vi "Simulation Interface.vi"(8 "error in (no error)":errorcluster) -> (0 "error out":errorcluster)   [LabVIEW 2017]
doc: "The simulated modules used to validate the Elevator Controller logic and algorithms."
uses:
  View Model/Controls/Interface.ctl
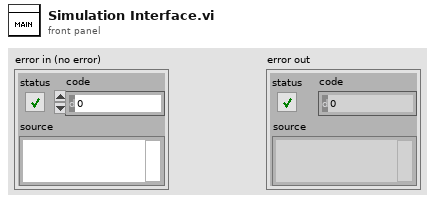
[diagram p1: front panel]
types:
  T1 = typedef "View Model.ctl" = cluster{"Shared Model":T2, "Error Model":T3, "Config Model":T4, "Control Model":T5}
  T2 = typedef "Shared Model.ctl" = cluster{"Stop":refnum<user-event>, "Stop DVR":refnum<data-value>}
  T3 = typedef "Error Model.ctl" = cluster{"Error":refnum<user-event>}
  T4 = typedef "Config Model.ctl" = cluster{"Data DVR":refnum<data-value>, "Config CMD":refnum<user-event>}
  T5 = typedef "Control Model.ctl" = cluster{"Location Change":refnum<user-event>, "Direction Change":refnum<user-event>, "Door Posit Change":refnum<user-event>, "Emergency Change":refnum<user-event>, "Status Change":refnum<user-event>, "Command":refnum<user-event>, "Overhaed DVR":refnum<data-value>}
  T6 = typedef "Interface.ctl" = enum16{"Simulated", "Physical"}
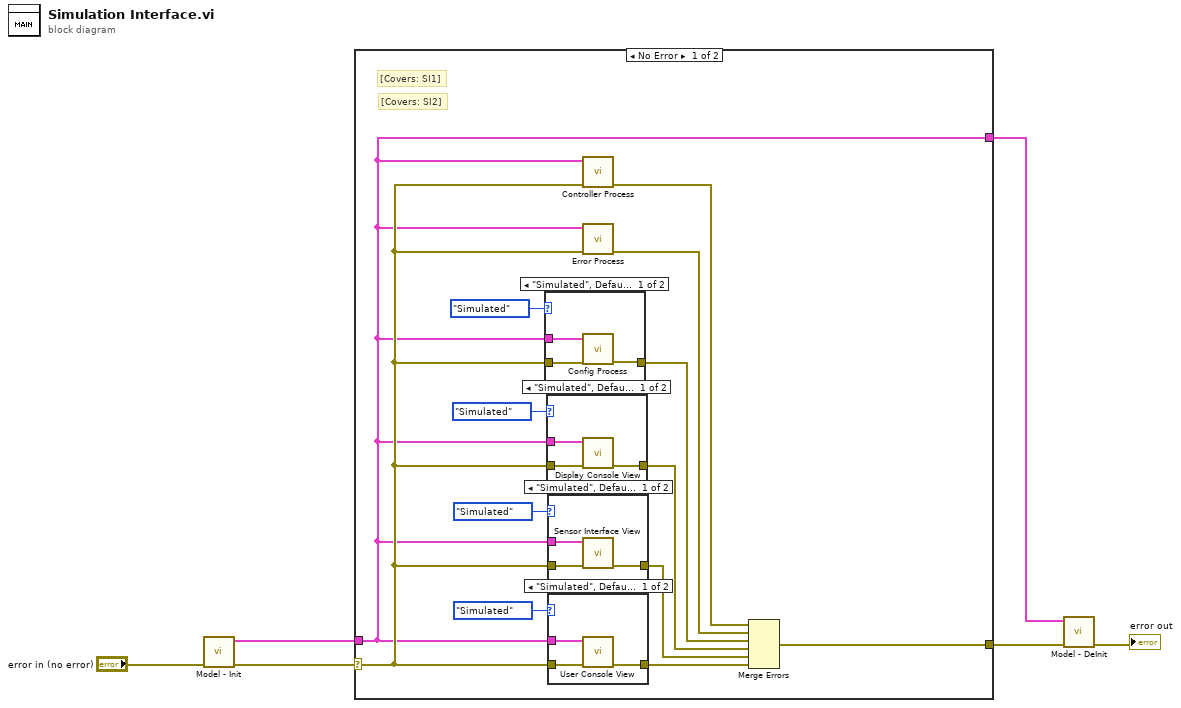
[diagram p0: block diagram]
diagram:
  n1 = call "Model - Init.vi"("error in (no error)"="error in (no error)") -> ("error out"=w4:errorcluster, "View Model"=w5:T1)  [unwired: 9 in]
  n2 = case shown="No Error" w4 {
    selector: w4 -> [w15 w37]
    tunnel: w5 -> [w7 w36]
    tunnel: [w8 w37] -> w3
    tunnel: [w7 w36] -> w1
    frame No Error {
      # "[Covers: SI2]"
      # "[Covers: SI1]"
      n3 = case shown="\"Simulated\", Default" Interface."Simulated" ("Interface") {
        tunnel: w7 -> [w21 _]
        tunnel: w15 -> [w22 w23]
        tunnel: [w20 w23] -> w11
        frame "Simulated", Default {
          n4 = call "Config Process.vi"("error in (no error)"=w22, "View Model"=w21) -> ("error out"=w20:errorcluster)  [unwired: 9 in]
        }
        frame "Physical" {
        }
      }
      n5 = case shown="\"Simulated\", Default" Interface."Simulated" ("Interface") {
        tunnel: w7 -> [w24 _]
        tunnel: w15 -> [w25 w27]
        tunnel: [w26 w27] -> w12
        frame "Simulated", Default {
          n6 = call "Display Console View.vi"("error in (no error)"=w25, "View Model"=w24) -> ("error out"=w26:errorcluster)  [unwired: 9 in]
        }
        frame "Physical" {
        }
      }
      n7 = case shown="\"Simulated\", Default" Interface."Simulated" ("Interface") {
        tunnel: w7 -> [w29 _]
        tunnel: w15 -> [w30 w31]
        tunnel: [w28 w31] -> w13
        frame "Simulated", Default {
          n8 = call "Sensor Interface View.vi"("error in (no error)"=w30, "View Model"=w29) -> ("error out"=w28:errorcluster)  [unwired: 9 in]
        }
        frame "Physical" {
        }
      }
      n9 = case shown="\"Simulated\", Default" Interface."Simulated" ("Interface") {
        tunnel: w7 -> [w34 _]
        tunnel: w15 -> [w33 w35]
        tunnel: [w32 w35] -> w14
        frame "Simulated", Default {
          n10 = call "User Console View.vi"("error in (no error)"=w33, "View Model"=w34) -> ("error out"=w32:errorcluster)  [unwired: 9 in]
        }
        frame "Physical" {
        }
      }
      n11 = call "Controller Process.vi"("error in (no error)"=w15, "View Model"=w7) -> ("error out"=w9:errorcluster)  [unwired: 9 in]
      n12 = call "Error Process.vi"("error in (no error)"=w15, "View Model"=w7) -> ("error out"=w10:errorcluster)  [unwired: 9 in]
      n13 = Merge Errors(w9, w10, w11, w12, w13, w14) -> (w8:errorcluster)
    }
    frame Error {
    }
  }
  n14 = call "Model - DeInit.vi"("error in (no error)"=w3, "View Model"=w1) -> ("error out"=→"error out":errorcluster)  [unwired: 9 in]
